vi "LimelightRead.vi"() -> (0 "tv":bool, 1 "camtran":dbl[](array[numeric]))   [LabVIEW 2018]
uses:
  <vilib>/Rock Robotics/Network Tables/NT Read Numeric Array.vi
  <vilib>/Rock Robotics/Network Tables/NT Read Number.vi
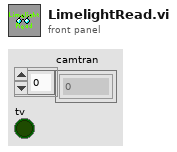
[diagram p1: front panel]
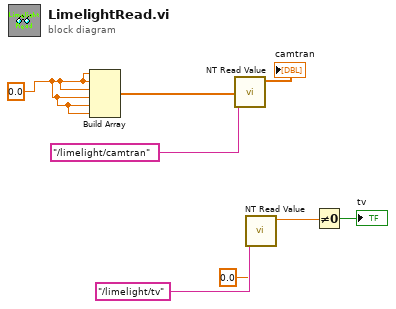
[diagram p0: block diagram]
diagram:
  w8 = 0.0
  n1 = Build Array(w8, w8, w8, w8, w8, w8) -> (w7:dbl[])
  n2 = call-poly <vilib>:"NT Read Value.vi"("Default Value"=w7, "Name"="/limelight/camtran") -> ("Numeric Array"=→"camtran":dbl[])  [unwired: 8 in, 1 out]
  n3 = call-poly <vilib>:"NT Read Value.vi"("Default Value"=0.0, "Name"="/limelight/tv") -> ("Numeric"=w2:dbl)  [unwired: 8 in, 1 out]
  n4 = Not Equal To 0?(x=w2) -> (x != 0?=→"tv":bool)
